vi "DSB Modulation Demo (Baseband-Sine) - Mozart.vi"() -> ()   [LabVIEW 2013]
uses:
  <vilib>/sound2/lvsound2.llb/Sound File Info (path).vi
  <vilib>/sound2/lvsound2.llb/Sound File Read Open.vi
  <vilib>/sound2/lvsound2.llb/Sound File Read (DBL).vi
  <vilib>/Waveform/WDTOps.llb/WDT Get Waveform Subset DBL.vi
  <vilib>/express/express analysis/Spectral/Block/exnSpectralBlock spectral measurements RMS poly.vi
  <vilib>/express/express analysis/Spectral/Block/exnSpectralBlock spectral measurements RMS DDT.vi
  <vilib>/express/express analysis/Spectral/Block/exnSpectralBlock spectral measurements power poly.vi
  <vilib>/express/express analysis/Spectral/Block/exnSpectralBlock spectral measurements power DDT.vi
  <vilib>/express/express analysis/Spectral/XNode/ExpressSpectralMeasurementsBlockNode.xnode
panel:
  out "Estimated Freq":dbl
  in  "Path":path=path "D:/wendy/study/2023-2024Spring/EE206lab/lab2/mozart.wav"
  in  "Duration":dbl=1000000.0 caption="Frequency"
  in  "Resample Rate":dbl=1000000.0 caption="Frequency"
  in  "?":enum32{"DSB FFT", "DSB Squared"}(tab)
  out "DSB FFT":dynamicdata(graph)
  out "DSB Squared":dynamicdata(graph)
  in  "WAV Sample Rate":dbl=44100.0 caption="dt"
  in  "LPF Cut-Off":dbl=10000.0 caption="Lower Cut-Off"
  in  "SNR (dB)":dbl(slide)=30.0 caption="Standard deviation" scale=-20.0..30.0
  out "Comparision":dynamicdata(graph)
  out "Baseband":dynamicdata(graph)
  out "DSB Wave":dynamicdata(graph)
  in  "Carrier Amp.":dbl=1.0 caption="Amplitude"
  in  "stop":bool
  in  "Frequency Offset":dbl(slide) scale=0.0..1000.0
  in  "Carrier Freq.":dbl=100000.0 caption="Frequency"
  # "DSB Modulation"
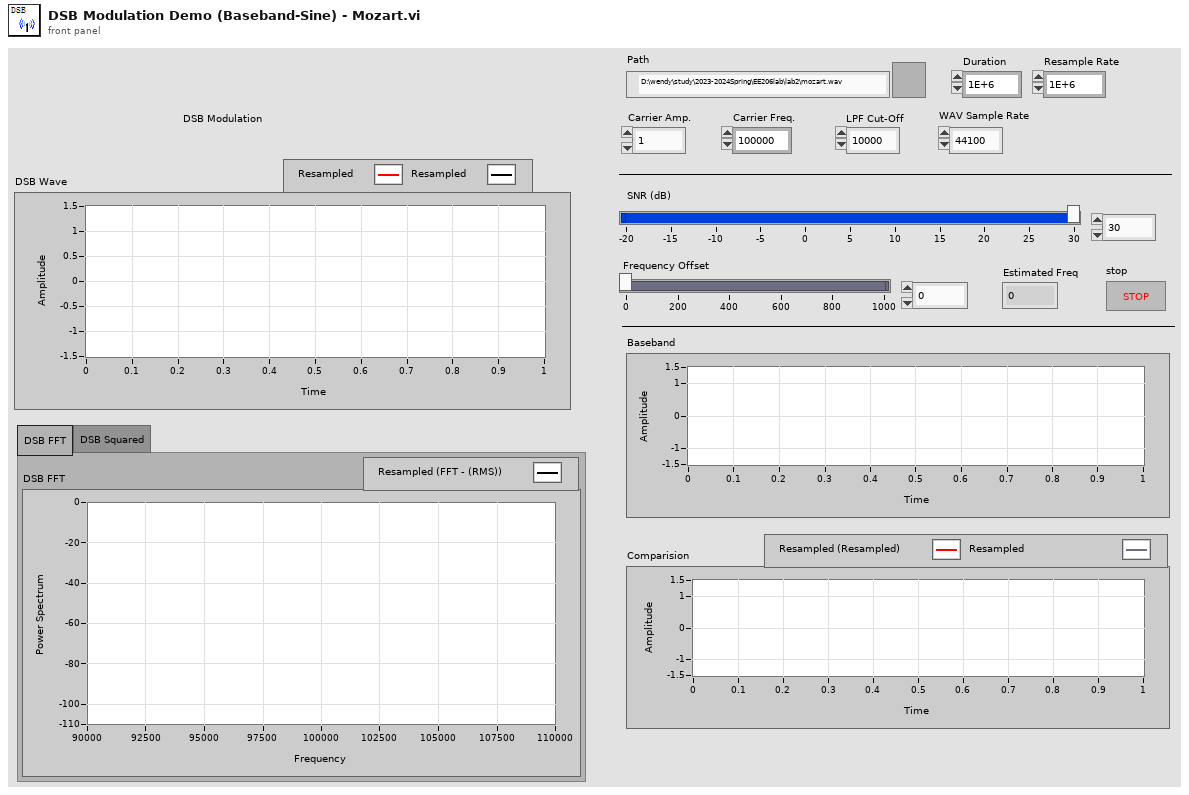
[diagram p1: front panel]
types:
  T1 = typedef "Sound File Refnum.ctl" = refnum<file>
  T2 = cluster{"averaging mode":u16, "weighting mode":u16, "number of averages":u32}
  T3 = cluster{"dB On (F)":bool, "unwrap phase (F)":bool, "convert to degree (F)":bool}
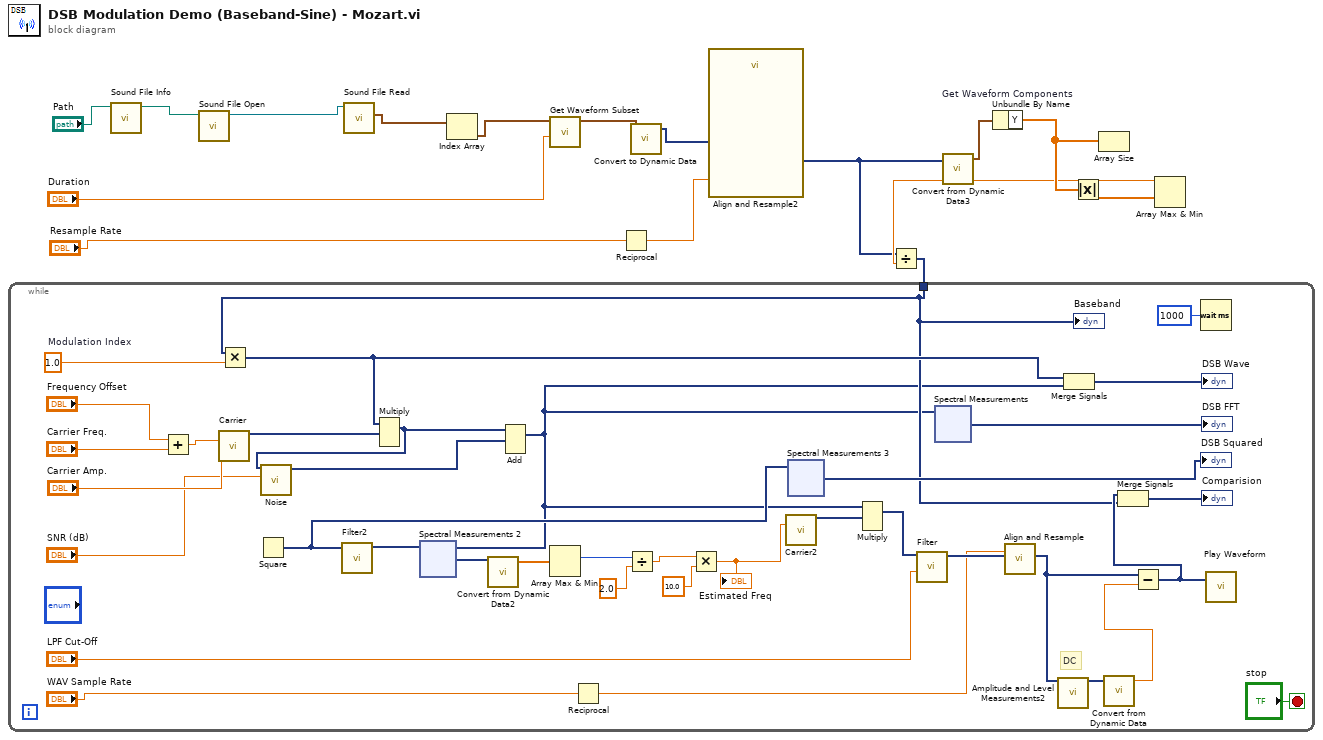
[diagram p0: block diagram]
diagram:
  n1 = call-poly <vilib>:"Sound File Info.vi"("path"="Path") -> ("path out"=w6:path)  [unwired: 7 in, 3 out]
  n2 = call-poly <vilib>:"Sound File Open.vi"("path"=w6) -> ("sound file refnum"=w15:T1)  [unwired: 9 in, 1 out]
  n3 = call-poly <vilib>:"Sound File Read.vi"("sound file refnum"=w15) -> ("data"=w14:waveform(dbl)[])  [unwired: 6 in, 4 out]
  n4 = Index Array "Index Array"(array=w14) -> (element=w13:waveform(dbl))  [unwired: 1 in]
  n5 = call-poly <vilib>:"Get Waveform Subset.vi"("duration"="Duration", "waveform in"=w13) -> ("waveform out"=w7:waveform(dbl))  [unwired: 4 in, 3 out]
  n6 = Reciprocal(x="Resample Rate") -> (1/x=w8:dbl)
  n7 = call "Convert to Dynamic Data"("Waveform"=w7) -> ("Dynamic Data Type"=w12:dynamicdata)  [unwired: 3 in]
  n8 = call "Align and Resample2"("dt"=w8, "Signals"=w12) -> ("Resampled Signals"=w5:dynamicdata)  [unwired: 7 in, 2 out]
  n9 = call "Convert from Dynamic Data3"("Dynamic Data Type"=w5) -> ("Waveform"=w4:waveform(dbl))  [unwired: 3 in]
  n10 = Unbundle By Name "Get Waveform Components"(w4) -> ("Y"=w11:dbl[])
  n11 = Absolute Value(x=w11) -> (abs(x)=w10:dbl[])
  n12 = Array Size(array=w11) -> ()  [unwired: 1 out]
  n13 = Array Max & Min(array=w10) -> (max value=w9:dbl)  [unwired: 3 out]
  n14 = Divide(x=w5, y=w9) -> (x/y=w1:dynamicdata)
  n15 = while {
    tunnel: w1 -> [w18]
    stop <- "stop" stop-if-true
    w47 = 1.0  # Modulation Index
    # "DC"
    n16 = Add(x="Frequency Offset", y="Carrier Freq.") -> (x+y=w46:dbl)
    n17 = call "Carrier"("Frequency"=w46, "Amplitude"="Carrier Amp.") -> ("Sine"=w44:dynamicdata)  [unwired: 12 in, 1 out]
    n18 = Multiply(x=w18, y=w47) -> (x*y=w43:dynamicdata)
    n19 = Multiply(1:w44, 2:w43) -> (0:w30:dynamicdata)  [unwired: 1 in, 1 out]
    n20 = call "Noise.vi"("AWGN (dB)"="SNR (dB)", "Dynamic Data"=w30) -> ("DC with Gaussian Noise"=w42:dynamicdata)  [unwired: 9 in]
    n21 = Add(1:w42, 2:w30) -> (0:w17:dynamicdata)  [unwired: 1 in, 1 out]
    n22 = Square(x=w17) -> (x^2=w29:dynamicdata)
    n23 = call "Filter2"("Signal"=w29) -> ("Filtered Signal"=w26:dynamicdata)  [unwired: 9 in, 1 out]
    n24 = xnode "Spectral Measurements 2"("Signals"=w26) -> ("Power Spectrum"=w25:dynamicdata)  [unwired: 1 in, 1 out]
    n25 = call "Convert from Dynamic Data2"("Dynamic Data Type"=w25) -> ("Array"=w24:dbl[])  [unwired: 3 in]
    n26 = Array Max & Min(array=w24) -> (max index (indices)=w23:i32)  [unwired: 3 out]
    n27 = Reciprocal(x="WAV Sample Rate") -> (1/x=w31:dbl)
    n28 = Divide(x=w23, y=2.0) -> (x/y=w21:dbl)
    n29 = Multiply(x=w21, y=10.0) -> (x*y=w19:dbl)
    "Estimated Freq" <- w19
    n30 = call "Carrier2"("Frequency"=w19) -> ("Sine"=w39:dynamicdata)  [unwired: 13 in, 1 out]
    n31 = xnode "Spectral Measurements 3"("Signals"=w29) -> ("FFT - (RMS)"=→"DSB Squared":dynamicdata)  [unwired: 2 in, 3 out]
    n32 = Multiply(1:w39, 2:w17) -> (0:w38:dynamicdata)  [unwired: 1 in, 1 out]
    n33 = call "Filter"("Lower Cut-Off"="LPF Cut-Off", "Signal"=w38) -> ("Filtered Signal"=w37:dynamicdata)  [unwired: 8 in, 1 out]
    n34 = xnode "Spectral Measurements"("Signals"=w17) -> ("FFT - (RMS)"=→"DSB FFT":dynamicdata)  [unwired: 2 in, 3 out]
    n35 = call "Align and Resample"("dt"=w31, "Signals"=w37) -> ("Resampled Signals"=w50:dynamicdata)  [unwired: 7 in, 2 out]
    n36 = call "Amplitude and Level Measurements2"("Signals"=w50) -> ("Mean (DC)"=w52:dynamicdata)  [unwired: 13 in, 1 out]
    n37 = Merge Signals(w43, w17) -> (→"DSB Wave":dynamicdata)
    n38 = call "Convert from Dynamic Data"("Dynamic Data Type"=w52) -> ("Scalar"=w49:dbl)  [unwired: 3 in]
    n39 = Subtract(x=w50, y=w49) -> (x-y=w35:dynamicdata)
    n40 = Merge Signals(w35, w18) -> (→"Comparision":dynamicdata)
    n41 = Wait (ms)(milliseconds to wait=u32 1000) -> ()  [unwired: 1 out]
    n42 = call "Play Waveform"("Data"=w35) -> ()  [unwired: 18 in, 1 out]
    "Baseband" <- w18
  }
